vi "Wire Probe.vi"(11 "channel":T1) -> (2 "Value String":string="See Channel Status Window for information.", 3 "Boolean":bool)   [LabVIEW 2017, in "Stream-t'WPI_EncoderType.ctl'.lvlib"]
uses:
  <extravilib>/ChannelInstances/Stream-t'WPI_EncoderType.ctl'.lvlib
  <extravilib>/ChannelInstances/Stream-t'WPI_EncoderType.ctl'/)Channel.ctl
  <vilib>/Rock Robotics/WPI/Encoder/WPI_EncoderType.ctl
  <extravilib>/ChannelInstances/Stream-t'WPI_EncoderType.ctl'/ChannelOp.ctl
  <extravilib>/ChannelInstances/Stream-t'WPI_EncoderType.ctl'/StreamData.lvclass
panel:
  in  "Default Text":string="* If the diagram containing this channel wire has already activated, the channel probe will open immediately.\n\n* Otherwise, the channel probe will open when the diagram that contains this wire probe next activates. To probe a channel from the very beginning of its lifetime, set a wire probe on the channel wire at the highest level diagram where branches from the writers and readers meet up. See \"Probing Channel Wires\" in the LabVIEW help for more information."
  out "Display":string="* If the diagram containing this channel wire has already activated, the channel probe will open immediately.\n\n* Otherwise, the channel probe will open when the diagram that contains this wire probe next activates. To probe a channel from the very beginning of its lifetime, set a wire probe on the channel wire at the highest level diagram where branches from the writers and readers meet up. See \"Probing Channel Wires\" in the LabVIEW help for more information."
  in  "pause on activation?":bool
  in  "Could Not Allocate Probe":string="Could not create probe because of low memory. Please free up memory so that LabVIEW may allocate a channel probe."
  in  "Mismatched Type":string="Could not create probe because of type mismatch. Please alert National Instruments about this error. Until this is repaired, channels of this kind cannot be probed."
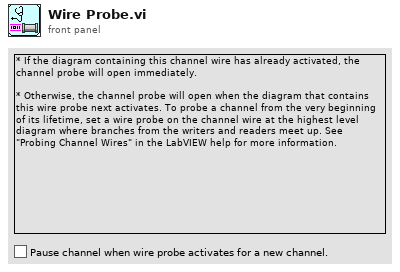
[diagram p1: front panel]
types:
  T1 = typedef "Stream-t'WPI_EncoderType.ctl'.lvlib/)Channel.ctl" = refnum<queue>
  T2 = typedef "Stream-t'WPI_EncoderType.ctl'.lvlib/ChannelOp.ctl" = enum16{"init", "write", "read", "probe"}
  T3 = enum32{"Invalid", "Standard", "Closed", "Hidden", "Minimized", "Maximized"}
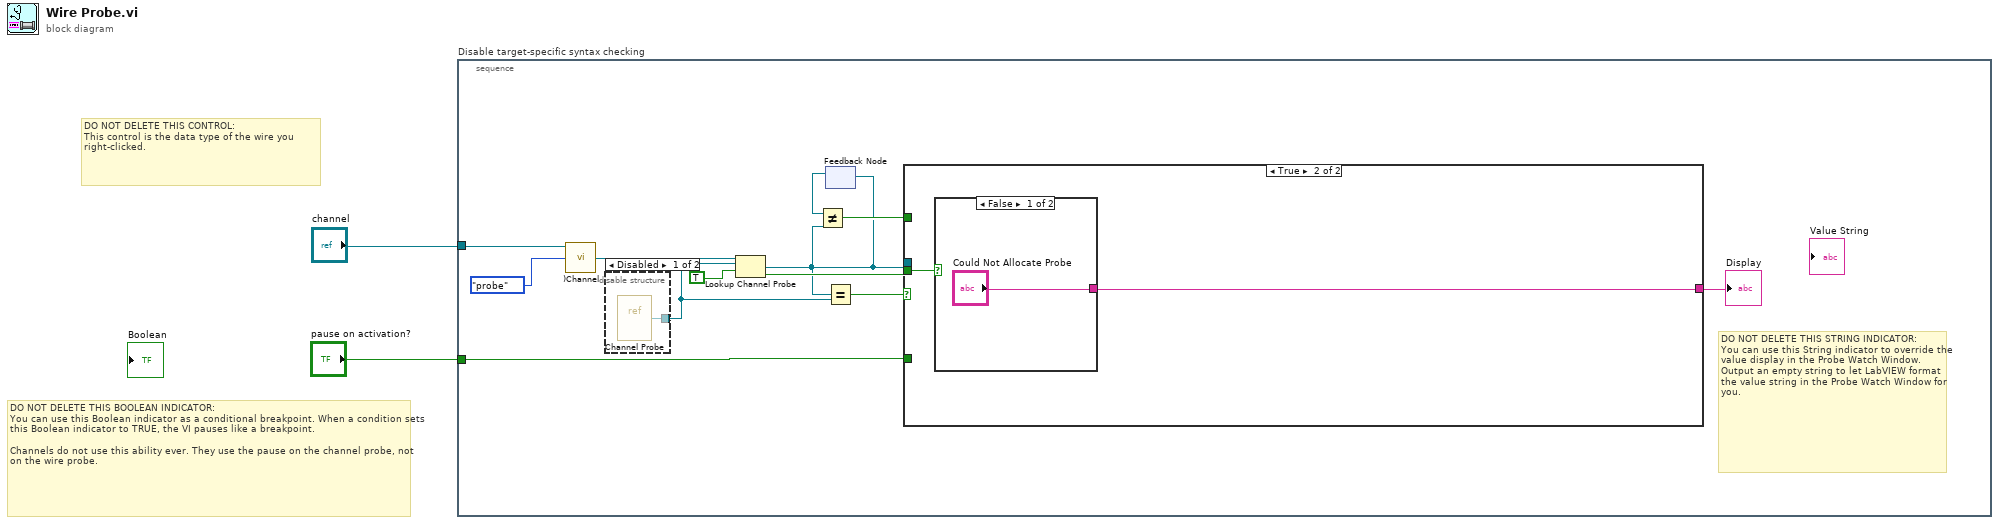
[diagram p0: block diagram]
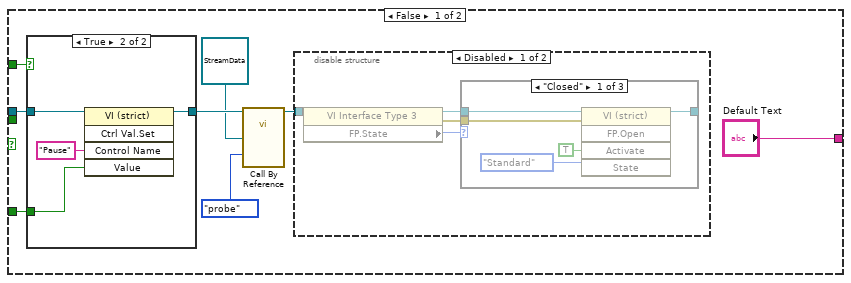
[diagram p3: hidden frame]
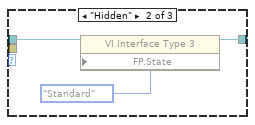
[diagram p4: hidden frame]
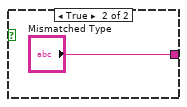
[diagram p8: hidden frame]
diagram:
  # "DO NOT DELETE THIS BOOLEAN INDICATOR: \nYou can use this Boolean indicator as a conditional breakpoint. When a condition sets this Boolean indicator to TRUE, the VI pauses like a breakpoint.\n\nChannels do not use this ability ever. They use the pause on the channel probe, not on the wire probe."
  # "DO NOT DELETE THIS CONTROL: \nThis control is the data type of the wire you right-clicked."
  n1 = stacked-sequence "Disable target-specific syntax checking" {
    tunnel: "pause on activation?" -> [w6]
    tunnel: "channel" -> [w3]
    frame #0 {
      # "DO NOT DELETE THIS STRING INDICATOR: \nYou can use this String indicator to override the value display in the Probe Watch Window.  Output an empty string to let LabVIEW format the value string in the Probe Watch Window for you."
      n2 = call <extravilib>:")Channel.vi"("channel in"=w3, "channelOp"=ChannelOp."probe") -> ("This VI out"=w4:refnum<vi>)  [unwired: 6 in, 7 out]
      n3 = disable-structure shown="Disabled" {
        disable-tunnel: [w15 _] -> w7
        frame Disabled {
          n4 = vi-ref <extravilib>:"Channel Probe.vi"() -> (w15:refnum<vi>)
        }
        frame Enabled {
        }
      }
      n5 = Lookup Channel Probe(0:w4, 1:w7, 2:TRUE ("force create?")) -> (9:w9:refnum<vi>, 10:w12:bool)
      n6 = feedback #1() -> (w11:refnum<vi>)  [unwired: 1 in]
      n7 = Not Equal?(x=w11, y=w9) -> (x != y?=w10:bool)
      n8 = feedback-in #1(w9) -> ()
      n9 = Equal?(x=w9, y=w7) -> (x = y?=w13:bool)
      n10 = case shown="True" w13 {
        tunnel: w12 -> [_ w43]
        tunnel: ["Default Text" w42] -> w8
        tunnel: w9 -> [w23 _]
        tunnel: w6 -> [w22 _]
        tunnel: w10 -> [w21 _]
        frame False {
          n11 = case shown="True" w21 {
            tunnel: w23 -> [w37 w41]
            tunnel: w22 -> [_ w39]
            tunnel: [w37 w38] -> w20
            frame False {
            }
            frame True {
              n12 = invoke class="VI (strict)" method="Ctrl Val.Set"(reference=w41, "Control Name"="Pause", "Value"=w39) -> (reference out=w38:refnum<vi>)  [unwired: 2 in, 4 out]
            }
          }
          n13 = call-by-ref "?"(reference=w20, "channelOp"=ChannelOp."probe", "PipeData in"=refnum<class "StreamData.lvclass"> refnum) -> (reference out=w19:refnum<vi>)  [unwired: 2 in, 2 out]
          n14 = disable-structure shown="Disabled" {
            disable-tunnel: w19 -> [w24 _]
            frame Disabled {
              n15 = property class="VI Interface Type 3"(reference=w24) -> (reference out=w25:refnum<vi>, error out=w26:errorcluster, "FP.State"=w27:T3)  [unwired: 1 in]
              n16 = case shown="\"Closed\"" w27 {
                tunnel: w26 -> [w31 _ _]
                tunnel: w25 -> [w32 w35 w36]
                tunnel: [w28 w34 w36] -> _
                frame "Closed" {
                  n17 = invoke class="VI (strict)" method="FP.Open"(reference=w32, error in=w31, "Activate"=TRUE ("Activate?"), "State"=T3."Standard") -> (reference out=w28:refnum<vi>)  [unwired: 1 in, 4 out]
                }
                frame "Hidden" {
                  n18 = property class="VI Interface Type 3"(reference=w35, "FP.State"=T3."Standard" ("Front Panel Window:State")) -> (reference out=w34:refnum<vi>)  [unwired: 1 in, 1 out]
                }
                frame Default {
                }
              }
            }
            frame Enabled {
            }
          }
        }
        frame True {
          n19 = case shown="False" w43 {
            tunnel: ["Could Not Allocate Probe" "Mismatched Type"] -> w42
            frame False {
            }
            frame True {
            }
          }
        }
      }
      "Display" <- w8
    }
  }
